vi "A-GAIN lookup table.vi"(10 "Enum":T1) -> (2 "Gain Value":i32)   [LabVIEW 2014, in "AMS TS3472 Light Sensor.lvlib" / "AMS TCS3472.lvclass"]
uses:
  AMS TCS3472.lvclass
  A-GAIN lookup table.ctl
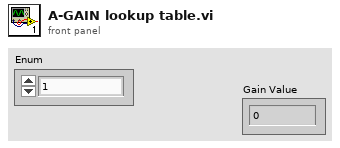
[diagram p1: front panel]
types:
  T1 = typedef "AMS TS3472 Light Sensor.lvlib/AMS TCS3472.lvclass/A-GAIN lookup table.ctl" = enum16{"1", "4", "16", "60"}
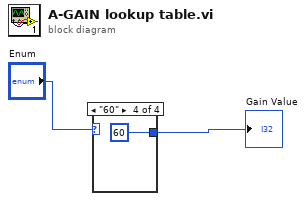
[diagram p0: block diagram]
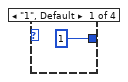
[diagram p2: hidden frame]
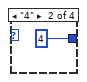
[diagram p3: hidden frame]
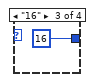
[diagram p4: hidden frame]
diagram:
  n1 = case shown="\"60\"" "Enum" {
    tunnel: [1 4 16 60] -> w2
    frame "1", Default {
    }
    frame "4" {
    }
    frame "16" {
    }
    frame "60" {
    }
  }
  "Gain Value" <- w2
